vi "Write Client.vi"(8 "error in (no error)":errorcluster, 10 "Client":string, 11 "RxTx in":refnum<class "RxTx.lvclass">) -> (0 "error out":errorcluster, 3 "RxTx out":refnum<class "RxTx.lvclass">)   [LabVIEW 2018, in "RxTx.lvclass"]
uses:
  RxTx.lvclass
  RxTx.lvclass/RxTx.ctl
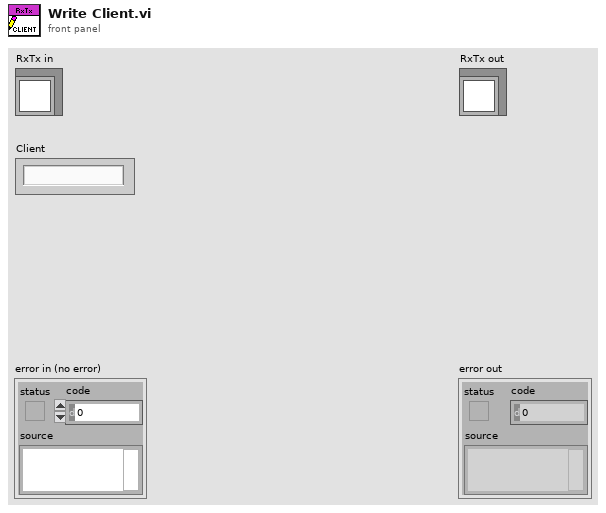
[diagram p1: front panel]
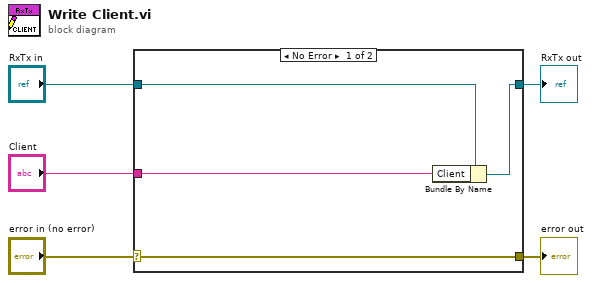
[diagram p0: block diagram]
diagram:
  n1 = case shown="No Error" "error in (no error)" {
    selector: "error in (no error)" -> [w9 w10]
    tunnel: [w9 w10] -> w4
    tunnel: [w7 w11] -> w2
    tunnel: "RxTx in" -> [w8 w11]
    tunnel: "Client" -> [w6 _]
    frame No Error {
      n2 = Bundle By Name(cluster=w8, "Client"=w6) -> (w7:refnum<class "RxTx.lvclass">)
    }
    frame Error {
    }
  }
  "error out" <- w4
  "RxTx out" <- w2
